vi "increment shared memory pointer.vi"(8 "Increment value":u64=8, 11 "Shared Memory PTR in":u64) -> (3 "Shared Memory PTR out":u64)   [LabVIEW 2018, in "linuxSharedMemory.lvlib"]
uses:
  linuxSharedMemory.lvlib
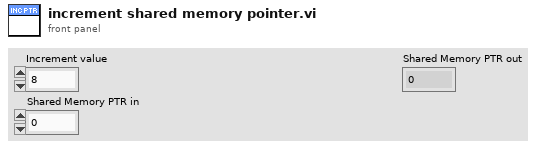
[diagram p1: front panel]
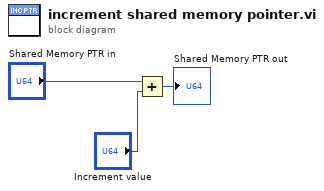
[diagram p0: block diagram]
diagram:
  n1 = Add(x="Shared Memory PTR in", y="Increment value") -> (x+y=→"Shared Memory PTR out":u64)
